vi "Enqueue Read-OFF.vi"(8 "Error In":errorcluster, 11 "Name":string) -> (0 "Error Out":errorcluster, 2 "Data":variant)   [LabVIEW 2019, in "SR_2000.lvlib"]
uses:
  SR_2000.lvlib
  Queue/Queue.lvlib
  Data Error Notifier/Data and Error Notifier.lvlib
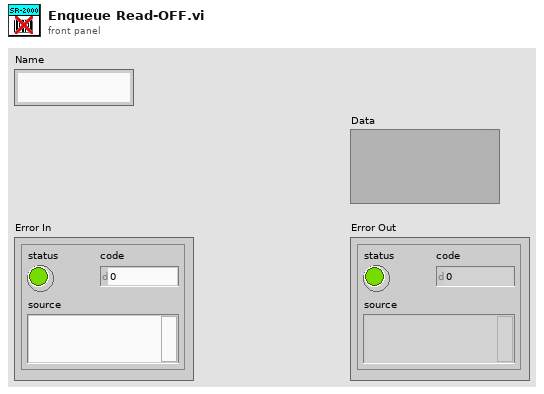
[diagram p1: front panel]
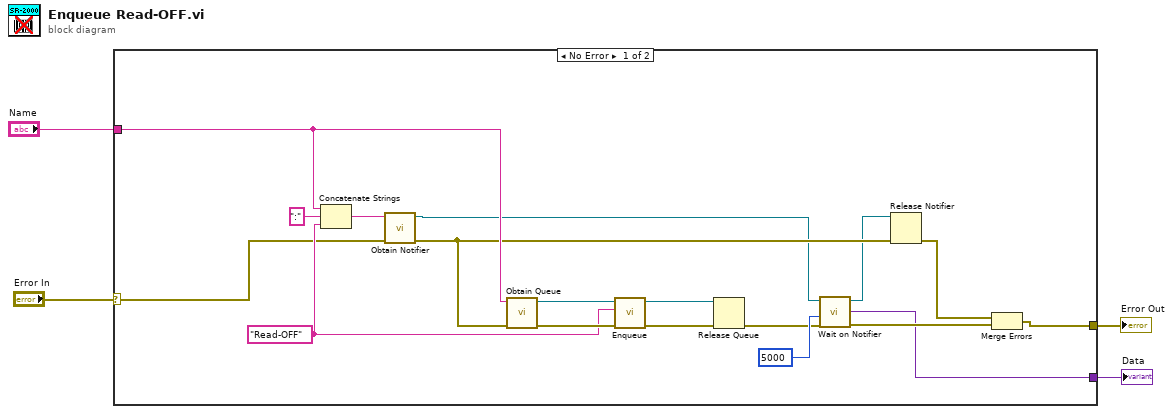
[diagram p0: block diagram]
diagram:
  n1 = case shown="No Error" "Error In" {
    selector: "Error In" -> [w12 w23]
    tunnel: [w14 w23] -> w3
    tunnel: "Name" -> [w21 _]
    tunnel: [w5 _] -> w1
    frame No Error {
      w19 = "Read-OFF" ("Message")
      n2 = Concatenate Strings(w21, ":" ("string"), w19) -> (w13:string)
      n3 = call "Obtain Notifier.vi"("Error In"=w12, "Name"=w13) -> ("Error Out"=w11:errorcluster, "notifier out"=w10:refnum<notifier>)  [unwired: 8 in]
      n4 = call "Obtain Queue.vi"("Error In"=w11, "Name"=w21) -> ("Error Out"=w22:errorcluster, "queue out"=w17:refnum<queue>)  [unwired: 8 in]
      n5 = call "Enqueue.vi"("Error In"=w22, "Message"=w19, "queue in"=w17) -> ("Error Out"=w18:errorcluster, "queue out"=w16:refnum<queue>)  [unwired: 7 in]
      n6 = Release Queue(queue=w16, error in (no error)=w18) -> (error out=w8:errorcluster)  [unwired: 1 in, 2 out]
      n7 = call "Wait on Notifier.vi"("Error In"=w8, "timeout in ms (-1)"=5000, "notifier in"=w10) -> ("Error Out"=w6:errorcluster, "Data"=w5:variant, "notifier out"=w7:refnum<notifier>)  [unwired: 6 in]
      n8 = Release Notifier(notifier=w7, error in (no error)=w11) -> (error out=w15:errorcluster)  [unwired: 1 in, 2 out]
      n9 = Merge Errors(w15, w6) -> (w14:errorcluster)
    }
    frame Error {
    }
  }
  "Error Out" <- w3
  "Data" <- w1
